vi "joystick to velocity.vi"(9 "max velocity":dbl, 11 "joystick main":dbl) -> (1 "lower bound":dbl, 2 "upper bound":dbl, 3 "Velocity":dbl)   [LabVIEW 2012]
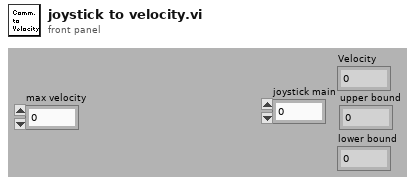
[diagram p1: front panel]
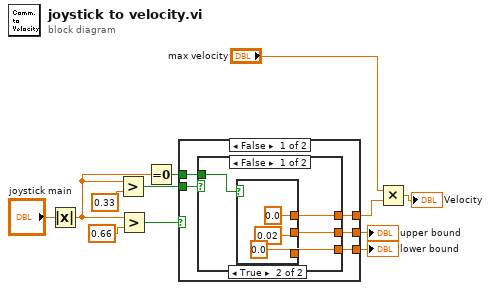
[diagram p0: block diagram]
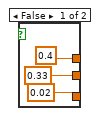
[diagram p2: hidden frame]
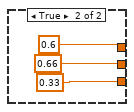
[diagram p3: hidden frame]
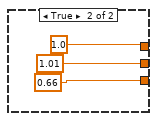
[diagram p4: hidden frame]
diagram:
  n1 = Absolute Value(x="joystick main") -> (abs(x)=w3:dbl)
  n2 = Greater?(x=w3, y=0.33) -> (0:w10:bool)
  n3 = Greater?(x=w3, y=0.66 ("Numeric")) -> (0:w12:bool)
  n4 = Equal To 0?(x=w3) -> (x = 0?=w2:bool)
  n5 = case shown="False" w12 {
    tunnel: w10 -> [w17 _]
    tunnel: [w16 1.0 ("y")] -> w8
    tunnel: [w15 1.01 ("y")] -> w5
    tunnel: [w14 0.66 ("y")] -> w4
    tunnel: w2 -> [w13 _]
    frame False {
      n6 = case shown="False" w17 {
        tunnel: [w19 0.6 ("y")] -> w16
        tunnel: [w20 0.66 ("y")] -> w15
        tunnel: [w21 0.33 ("y")] -> w14
        tunnel: w13 -> [w18 _]
        frame False {
          n7 = case shown="True" w18 {
            tunnel: [0.02 ("y") 0.0 ("y")] -> w21
            tunnel: [0.33 ("y") 0.02 ("y")] -> w20
            tunnel: [0.4 ("y") 0.0 ("y")] -> w19
            frame False {
            }
            frame True {
            }
          }
        }
        frame True {
        }
      }
    }
    frame True {
    }
  }
  "upper bound" <- w5
  "lower bound" <- w4
  n8 = Multiply(x="max velocity", y=w8) -> (x*y=→"Velocity":dbl)
